vi "LAS-CTS_NDFilterScanBackwards.vi"() -> ()   [LabVIEW 2024]
uses:
  <vilib>/httpClient/LabVIEWHTTPClient.lvlib
  <vilib>/Analysis/NI_AALBase.lvlib
panel:
  in  "Starting Position":i32
  out "Ion Current Chart":dbl(graph)
  out "Average Ion Current (pA)":dbl format="%.3g"
  in  "Ammeter Range":dbl(ring)=0.02 items=["20 mA"=0.02, "2 mA"=0.002, "200 uA"=0.0002, "20 uA"=2e-05, "2 uA"=2e-06, "200 nA"=2e-07, "20 nA"=2e-08, "2 nA"=2e-09, "200 pA"=2e-10, "20 pA"=2e-11]
  in  "Keithly":refnum<visa-resource-name>
  out "Laser Energy Chart":dbl(graph)
  out "Average Laser Energy (uJ)":dbl format="%.3g"
  out "ND Filter Position":i32
  in  "file path (use dialog)":path
  in  "Step Size":i32
  in  "ND Filter":refnum<visa-resource-name>
  in  "Number of Pulses":i32
  out "number of measurements":i32
  out "Laser Energy (uJ)":dbl
  in  "Energy Meter":refnum<visa-resource-name>
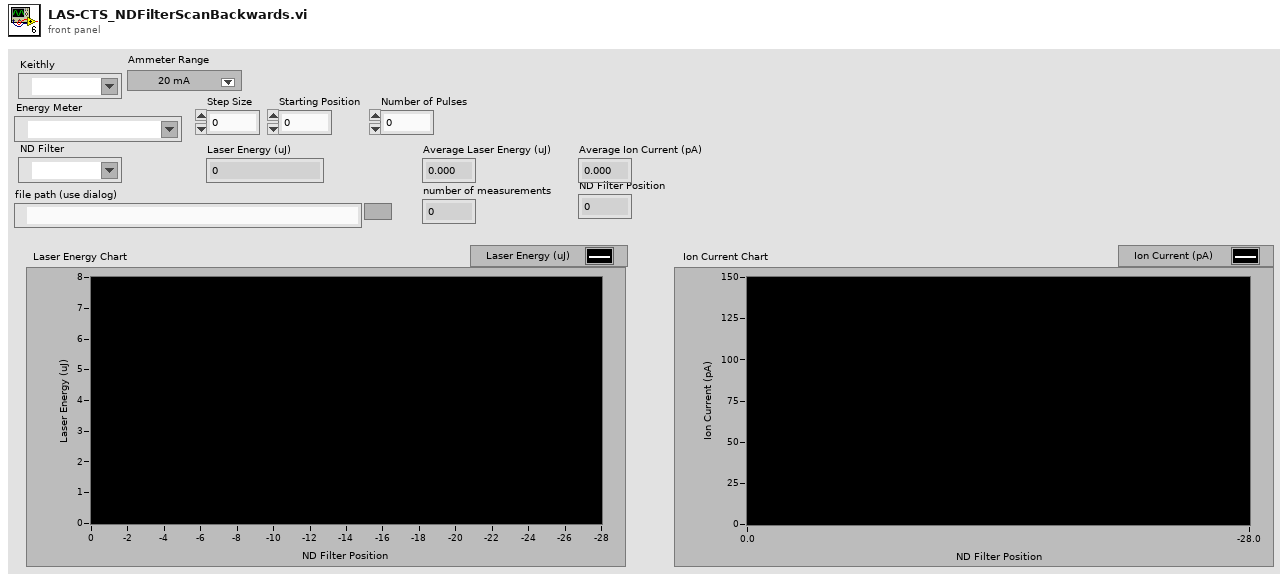
[diagram p1: front panel]
types:
  T1 = enum16{"open", "replace", "create", "open or create", "replace or create", "replace or create with confirmation"}
  T2 = typedef "LabVIEWHTTPClient.lvlib/ClientHandle.ctl" = refnum<k1>
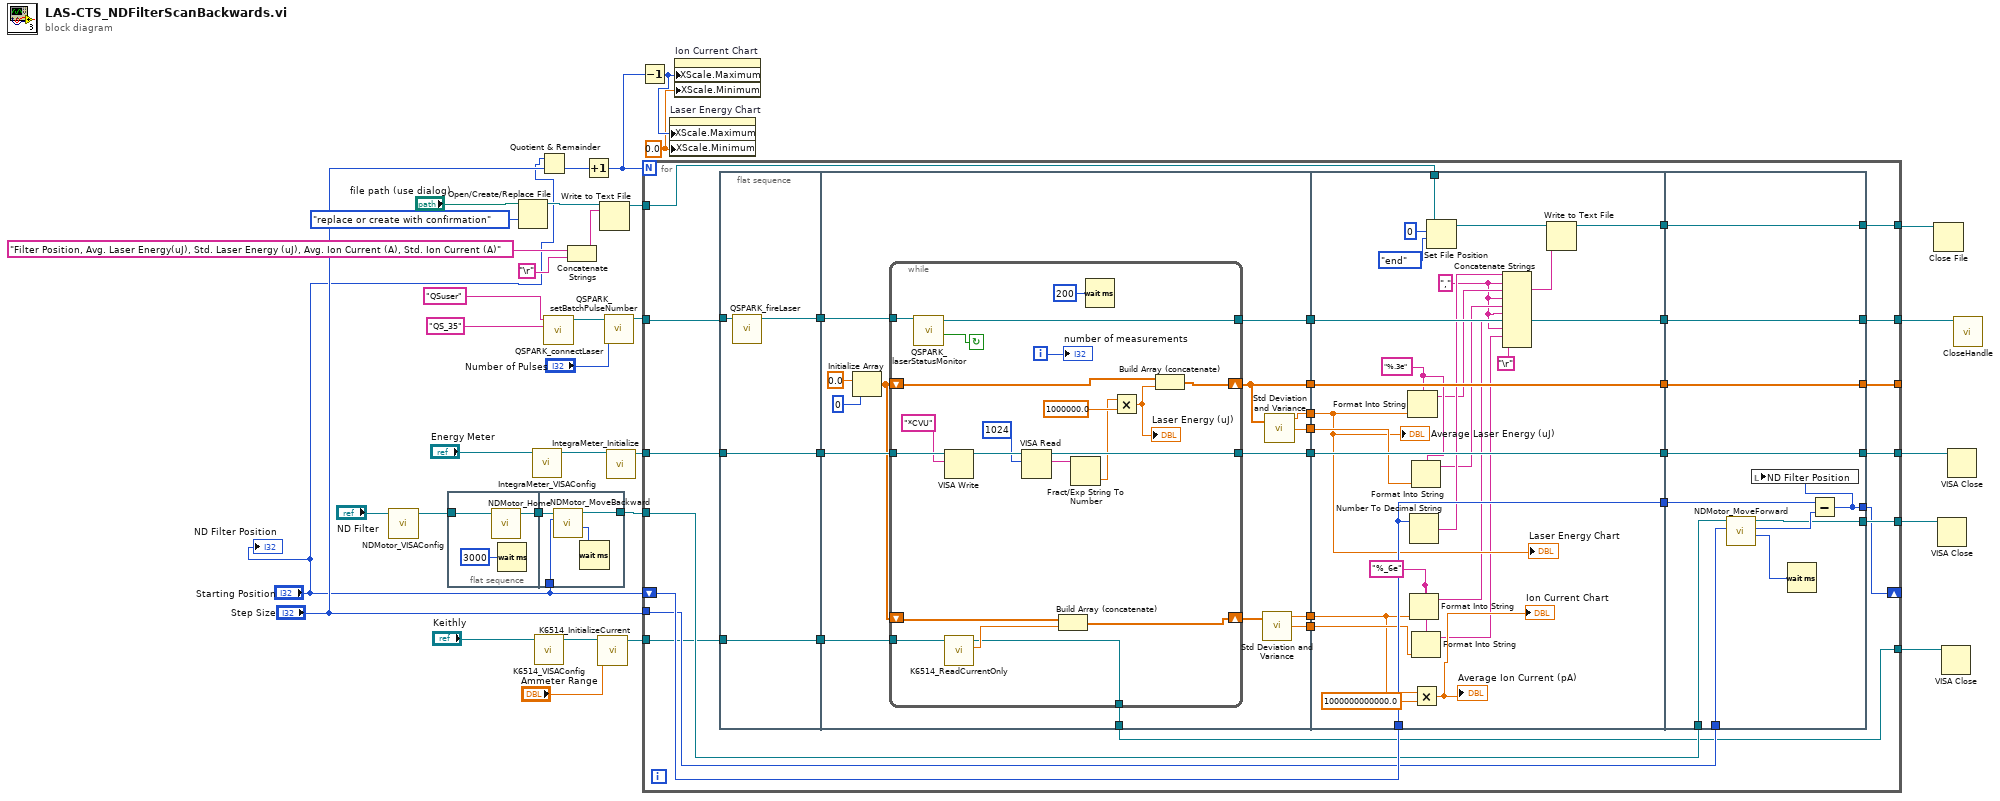
[diagram p0: block diagram]
diagram:
  w7 = 0.0 ("X Scale.Range:Minimum")
  n1 = call "NDMotor_VISAConfig.vi"("VISA resource name"="ND Filter") -> ("reference out"=w23:refnum<visa-resource-name>)  [unwired: 9 in, 1 out]
  n2 = flat-sequence {
    tunnel: w23 -> [w37]
    tunnel: [w36] -> w3
    tunnel: w3 -> [w41]
    tunnel: [w40] -> w2
    tunnel: "Starting Position" -> [w38]
    frame #0 {
      n3 = call "NDMotor_Home.vi"("VISA resource name"=w37) -> ("VISA resource name out"=w36:refnum<visa-resource-name>)  [unwired: 9 in, 1 out]
      n4 = Wait (ms)(milliseconds to wait=u32 3000) -> ()  [unwired: 1 out]
    }
    frame #1 {
      n5 = call "NDMotor_MoveBackward.vi"("Steps"=w38, "VISA resource name"=w41) -> ("move time (ms)"=w39:i32, "VISA resource name out"=w40:refnum<visa-resource-name>)  [unwired: 6 in, 2 out]
      n6 = Wait (ms)(milliseconds to wait=w39) -> ()  [unwired: 1 out]
    }
  }
  n7 = Open/Create/Replace File(file path (use dialog)="file path (use dialog)", operation (0:open)=T1."replace or create with confirmation") -> (refnum out=w17:refnum<file>)  [unwired: 4 in, 2 out]
  n8 = call "IntegraMeter_VISAConfig.vi"("VISA resource name"="Energy Meter") -> ("reference out"=w34:refnum<visa-resource-name>)  [unwired: 9 in, 1 out]
  n9 = call "K6514_VISAConfig.vi"("VISA resource name"="Keithly") -> ("reference out"=w12:refnum<visa-resource-name>)  [unwired: 9 in, 1 out]
  n10 = Quotient & Remainder(x="Starting Position", y="Step Size") -> (floor(x/y)=w6:i32)  [unwired: 1 out]
  n11 = call "QSPARK_connectLaser.vi"("password"="QS_35", "username"="QSuser") -> ("client handle out"=w27:T2)  [unwired: 9 in]
  n12 = Concatenate Strings("Filter Position, Avg. Laser Energy(uJ), Std. Laser Energy (uJ), Avg. Ion Current (A), Std. Ion Current (A)" ("text"), "\r") -> (w20:string)
  n13 = Increment(x=w6) -> (x+1=w4:i32)
  n14 = call "K6514_InitializeCurrent.vi"("Range"="Ammeter Range", "VISA resource name"=w12) -> ("VISA resource name out"=w10:refnum<visa-resource-name>)  [unwired: 8 in, 1 out]
  n15 = Write to Text File(file (use dialog)=w17, text=w20) -> (refnum out=w19:refnum<file>)  [unwired: 2 in, 2 out]
  n16 = call "QSPARK_setBatchPulseNumber.vi"("Number of Pulses"="Number of Pulses", "client handle"=w27) -> ("client handle out"=w30:T2)  [unwired: 9 in]
  n17 = call "IntegraMeter_Initialize.vi"("VISA resource name"=w34) -> ("VISA resource name out"=w32:refnum<visa-resource-name>)  [unwired: 9 in, 1 out]
  n18 = Decrement(x=w4) -> (x-1=w8:i32)
  n19 = for {
    N: w4 -> [_]
    tunnel: [w64] -> _
    tunnel: "Step Size" -> [w52]
    tunnel: w19 -> [w60]
    tunnel: w30 -> [w66]
    tunnel: [w65] -> w28
    tunnel: w32 -> [w68]
    tunnel: [w67] -> w31
    tunnel: w2 -> [w50]
    tunnel: [w59] -> w18
    shift-right: [w42] -> _
    shift-left: "Starting Position" -> [w58]
    tunnel: [w51] -> w14
    tunnel: w10 -> [w46]
    tunnel: [w43] -> w9
    n20 = flat-sequence {
      tunnel: [w74] -> w70
      tunnel: [w72] -> w69
      tunnel: w66 -> [w73]
      tunnel: w68 -> [w74]
      tunnel: [w71] -> w47
      tunnel: w46 -> [w71]
      tunnel: w70 -> [w89]
      tunnel: w69 -> [w87]
      tunnel: [w88] -> w63
      tunnel: [w86] -> w62
      tunnel: [w83] -> w61
      tunnel: [w82] -> w49
      tunnel: [w81] -> w48
      tunnel: w47 -> [w80]
      tunnel: [w77] -> w45
      tunnel: [w76] -> w44
      tunnel: [w75] -> w43
      tunnel: w63 -> [w135]
      tunnel: w62 -> [w134]
      tunnel: w61 -> [w133]
      tunnel: w60 -> [w130]
      tunnel: w58 -> [w126]
      tunnel: [w135] -> w57
      tunnel: [w134] -> w56
      tunnel: [w133] -> w55
      tunnel: [w128] -> w54
      tunnel: [w126] -> w53
      tunnel: w49 -> [w116]
      tunnel: w48 -> [w124]
      tunnel: w45 -> [w117]
      tunnel: w44 -> [w120]
      tunnel: [w137] -> w42
      tunnel: [w143] -> w59
      tunnel: [w144] -> w64
      tunnel: [w145] -> w65
      tunnel: [w146] -> w67
      tunnel: w57 -> [w146]
      tunnel: w56 -> [w145]
      tunnel: w55 -> [w144]
      tunnel: w54 -> [w143]
      tunnel: w53 -> [w141]
      tunnel: w52 -> [w140]
      tunnel: [w139] -> w51
      tunnel: w50 -> [w138]
      frame #0 {
        n21 = call "QSPARK_fireLaser.vi"("client handle"=w73) -> ("client handle out"=w72:T2)  [unwired: 10 in]
      }
      frame #1 {
        n22 = Initialize Array(0.0 ("element"), 0 ("dimension size")) -> (w79:dbl[])
        n23 = while {
          tunnel: w89 -> [w110]
          tunnel: [w108] -> w88
          tunnel: w87 -> [w103]
          tunnel: [w102] -> w86
          shift-right: [w99] -> w83
          shift-left: w79 -> [w100]
          tunnel: w80 -> [w91]
          shift-right: [w93] -> w78
          shift-left: w79 -> [w94]
          tunnel: [w90] -> w75
          i -> [w104]
          stop <- w101 continue-if-true
          n24 = call "QSPARK_laserStatusMonitor.vi"("client handle"=w103) -> ("laser on?"=w101:bool, "client handle out"=w102:T2)  [unwired: 8 in, 1 out]
          n25 = VISA Write(VISA resource name=w110, write buffer="*CVU") -> (VISA resource name out=w109:refnum<visa-resource-name>)  [unwired: 1 in, 2 out]
          n26 = call "K6514_ReadCurrentOnly.vi"("VISA resource name"=w91) -> ("Current (A)"=w92:dbl, "VISA resource name out"=w90:refnum<visa-resource-name>)  [unwired: 6 in, 2 out]
          n27 = VISA Read(VISA resource name=w109, byte count=u32 1024) -> (VISA resource name out=w108:refnum<visa-resource-name>, read buffer=w105:string)  [unwired: 1 in, 2 out]
          n28 = Build Array (concatenate)(w94, w92) -> (w93:dbl[])
          n29 = Fract/Exp String To Number(string=w105) -> (number=w96:dbl)  [unwired: 3 in, 1 out]
          n30 = Wait (ms)(milliseconds to wait=u32 200 ("millisecond multiple")) -> ()  [unwired: 1 out]
          n31 = Multiply(x=w96, y=1000000.0) -> (x*y=w95:dbl)
          "Laser Energy (uJ)" <- w95
          n32 = Build Array (concatenate)(w100, w95) -> (w99:dbl[])
          "number of measurements" <- w104
        }
        n33 = call <vilib>:"Std Deviation and Variance.vi"("X"=w78) -> ("mean"=w77:dbl, "standard deviation"=w76:dbl)  [unwired: 1 in, 1 out]
        n34 = call <vilib>:"Std Deviation and Variance.vi"("X"=w83) -> ("mean"=w82:dbl, "standard deviation"=w81:dbl)  [unwired: 1 in, 1 out]
      }
      frame #2 {
        w119 = "%_6e" ("format string")
        w112 = "," ("string")
        w125 = "%.3e" ("format string")
        n35 = Format Into String(format string=w125, w116) -> (resulting string=w122:string)  [unwired: 2 in, 1 out]
        n36 = Number To Decimal String(number=w126) -> (decimal integer string=w123:string)  [unwired: 1 in]
        n37 = Format Into String(format string=w119, w117) -> (resulting string=w114:string)  [unwired: 2 in, 1 out]
        n38 = Format Into String(format string=w125, w124) -> (resulting string=w121:string)  [unwired: 2 in, 1 out]
        n39 = Format Into String(format string=w119, w120) -> (resulting string=w113:string)  [unwired: 2 in, 1 out]
        n40 = Multiply(x=w117, y=1000000000000.0) -> (x*y=→"Average Ion Current (pA)" →"Ion Current Chart":dbl)
        n41 = Set File Position(offset (in bytes) (0)=i64 0, refnum=w130, from (0:start)=enum16{"start", "end", "current"}."end") -> (refnum out=w129:refnum<file>)  [unwired: 1 in, 1 out]
        n42 = Concatenate Strings(w123, w112, w122, w112, w121, w112, w114, w112, w113, "\r") -> (w127:string)
        n43 = Write to Text File(file (use dialog)=w129, text=w127) -> (refnum out=w128:refnum<file>)  [unwired: 2 in, 2 out]
        "Average Laser Energy (uJ)" <- w116
        "Laser Energy Chart" <- w116
      }
      frame #3 {
        n44 = call "NDMotor_MoveForward.vi"("Steps"=w140, "VISA resource name"=w138) -> ("move time (ms)"=w136:i32, "steps"=w142:i32, "VISA resource name out"=w139:refnum<visa-resource-name>)  [unwired: 6 in, 1 out]
        n45 = Wait (ms)(milliseconds to wait=w136) -> ()  [unwired: 1 out]
        n46 = Subtract(x=w141, y=w142) -> (x-y=w137:i32)
        n47 = local write "ND Filter Position"(w137) -> ()
      }
    }
  }
  n48 = property on="Laser Energy Chart" class="WFChart (strict)"("XScale.Maximum"=w8, "XScale.Minimum"=w7) -> ()  [unwired: 2 in, 2 out]
  n49 = property on="Ion Current Chart" class="WFChart (strict)"("XScale.Maximum"=w8, "XScale.Minimum"=w7) -> ()  [unwired: 2 in, 2 out]
  n50 = Close File(refnum=w18) -> ()  [unwired: 1 in, 2 out]
  n51 = VISA Close(VISA resource name=w14) -> ()  [unwired: 1 in, 1 out]
  n52 = VISA Close(VISA resource name=w9) -> ()  [unwired: 1 in, 1 out]
  n53 = VISA Close(VISA resource name=w31) -> ()  [unwired: 1 in, 1 out]
  n54 = call <vilib>:"CloseHandle.vi"("client handle"=w28) -> ()  [unwired: 14 in, 1 out]
  "ND Filter Position" <- "Starting Position"
